vi "FlipSignsForDivSub.vi"(2 "RHS":string, 3 "operation":string) -> (1 "RHS fixed":string)   [LabVIEW 2012]
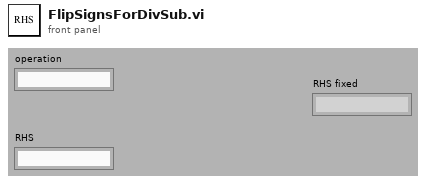
[diagram p1: front panel]
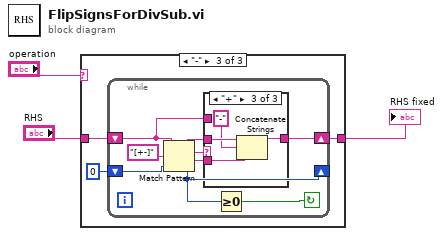
[diagram p0: block diagram]
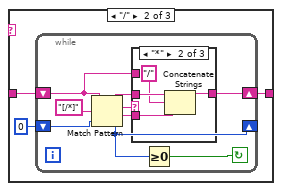
[diagram p3: hidden frame]
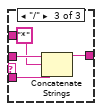
[diagram p5: hidden frame]
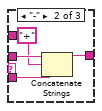
[diagram p7: hidden frame]
diagram:
  n1 = case shown="\"-\"" "operation" {
    tunnel: "RHS" -> [w4 w7 w28]
    tunnel: [w4 w6 w27] -> w1
    frame Default {
    }
    frame "/" {
      n2 = while {
        shift-right: [w12] -> w6
        shift-left: w7 -> [w11]
        shift-right: [w8] -> _
        shift-left: 0 ("offset past match") -> [w9]
        stop <- w10 continue-if-true
        n3 = Match Pattern(string=w11, regular expression="[/*]", offset (0)=w9) -> (before substring=w14:string, match substring=w15:string, after substring=w13:string, offset past match=w8:i32)
        n4 = case shown="\"*\"" w15 {
          tunnel: w14 -> [_ w21 w25]
          tunnel: w13 -> [_ w20 w24]
          tunnel: [w17 w18 w22] -> w12
          tunnel: w11 -> [w17 _ _]
          frame Default {
          }
          frame "*" {
            n5 = Concatenate Strings(w21, "/", w20) -> (w18:string)
          }
          frame "/" {
            n6 = Concatenate Strings(w25, "*", w24) -> (w22:string)
          }
        }
        n7 = Greater Or Equal To 0?(x=w8) -> (x >= 0?=w10:bool)
      }
    }
    frame "-" {
      n8 = while {
        shift-right: [w33] -> w27
        shift-left: w28 -> [w32]
        shift-right: [w29] -> _
        shift-left: 0 ("offset past match") -> [w30]
        stop <- w31 continue-if-true
        n9 = Match Pattern(string=w32, regular expression="[+-]", offset (0)=w30) -> (before substring=w35:string, match substring=w36:string, after substring=w34:string, offset past match=w29:i32)
        n10 = case shown="\"+\"" w36 {
          tunnel: w35 -> [_ w42 w46]
          tunnel: w34 -> [_ w41 w45]
          tunnel: [w38 w39 w43] -> w33
          tunnel: w32 -> [w38 _ _]
          frame Default {
          }
          frame "-" {
            n11 = Concatenate Strings(w42, "+", w41) -> (w39:string)
          }
          frame "+" {
            n12 = Concatenate Strings(w46, "-", w45) -> (w43:string)
          }
        }
        n13 = Greater Or Equal To 0?(x=w29) -> (x >= 0?=w31:bool)
      }
    }
  }
  "RHS fixed" <- w1
